vi "Prima lezione.vi"(1 "Manopola":dbl(knob)=1.0 scale=0.0..10.0 scale format="%#_7g") -> (0 "Numeric":dbl)   [LabVIEW 2012]
panel:
  out "Waveform Chart":cluster{"number: 0 to 1":dbl, dbl}(graph)
  out "Number\n(0 to 1)":dbl
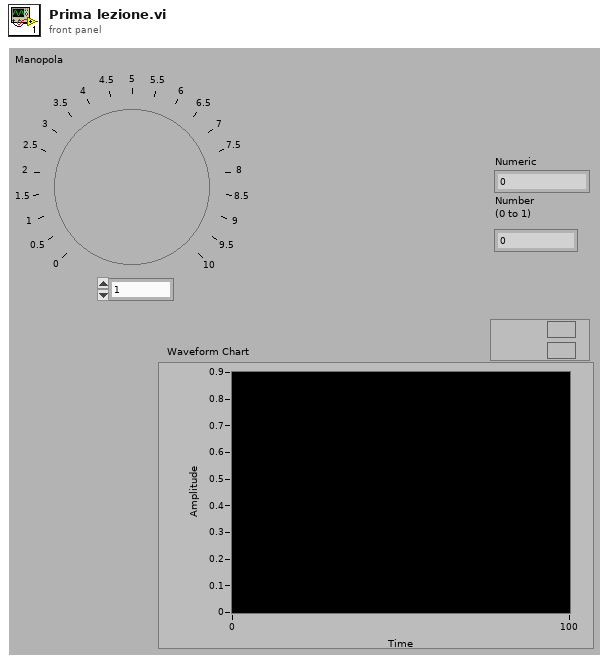
[diagram p1: front panel]
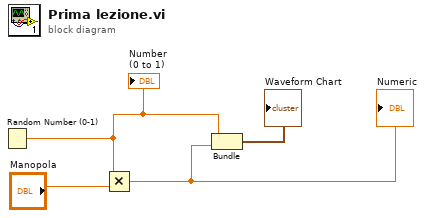
[diagram p0: block diagram]
diagram:
  n1 = Random Number (0-1)() -> (number: 0 to 1=w1:dbl)
  "Number\n(0 to 1)" <- w1
  n2 = Multiply(x=w1, y="Manopola") -> (x*y=w3:dbl)
  "Numeric" <- w3
  n3 = Bundle("number: 0 to 1"=w1, w3) -> (→"Waveform Chart":cluster{"number: 0 to 1":dbl, dbl})  [unwired: 1 in]
